vi "Stacking Commnd Sequencer.vi"(4 "Lifter Commands":T2, 5 "Command Series Start Index":i32, 6 "Wait Input":bool=TRUE, 7 "New Command Series":bool=TRUE, 8 "Set Motor Speed":dbl=0.25) -> (0 "Series Finished":bool, 1 "Grabber Solenoid":T1, 2 "Can Solenoid":T1, 3 "Motor Speed":dbl)   [LabVIEW 2014]
doc: "This VI runs a sequence of commands inputed into it. In order to use this properly, it is important to note that:\n -The Sequencer uses the lifter and when it reaches setpoints as the primary method of determining when to move on to another command\n - Currently, giving the lifter two or more identical setpoints in a row WILL cause it to FREEZE. DO NOT INPUT MULTIPLE IDENTICAL SETPOINTS. If you need the lifter to not move for a command, use the NO OP command.\n - The determination of when the command Sequence is completed is when there are four (4) NO OP commands in a row. IF YOU NEED MORE THAN THREE (3) NO OP COMMANDS,SEE ZEUS AND HE WILL CHANGE THE CODE.\n -If there is a wait time for that command, the wait time will OVERRIDE any \"Wait for Input\". In other words, you CANNOT use a WAIT command AND a WAIT TIME command in the same command."
uses:
  <vilib>/Rock Robotics/WPI/Solenoid/WPI_SolenoidValue.ctl
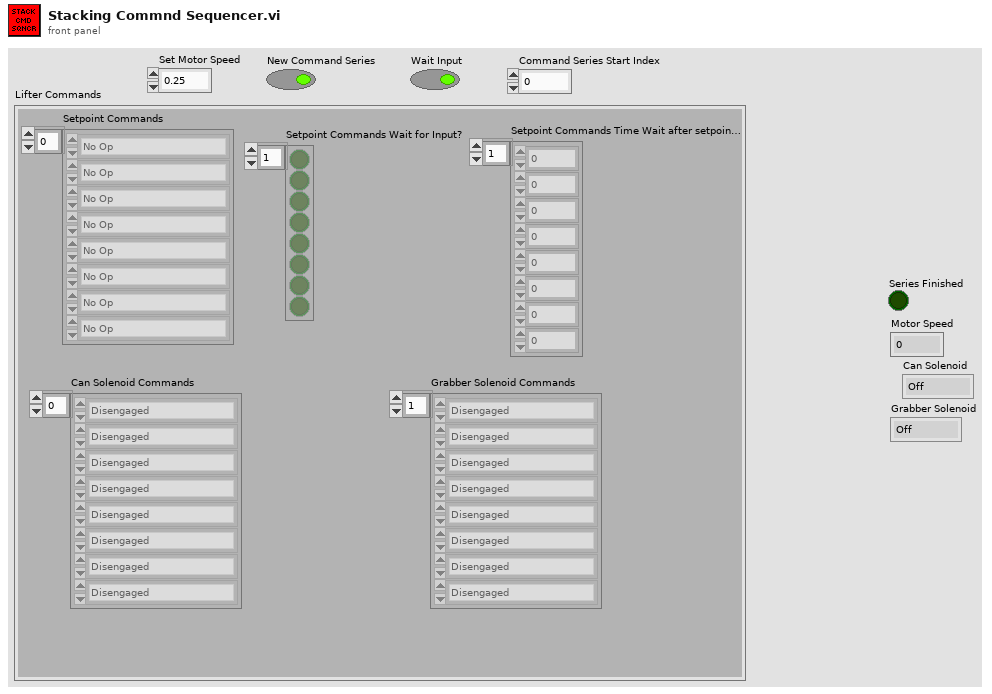
[diagram p1: front panel]
types:
  T1 = typedef "WPI_SolenoidValue.ctl" = enum16{"Off", "On", "Forward", "Reverse"}
  T2 = cluster{"Setpoint Commands":enum16{"No Op", "Setpoint 1", "Setpoint 2", "Setpoint 3", "Setpoint 4", "Setpoint 5"}[], "Setpoint Commands Wait for Input?":bool[], "Setpoint Commands Time Wait after setpoint reachd":i32[], "Can Solenoid Commands":enum16{"Disengaged", "Engaged"}[], "Grabber Solenoid Commands":enum16{"Disengaged", "Engaged"}[]}
  T3 = enum16{"No Op", "Setpoint 1", "Setpoint 2", "Setpoint 3", "Setpoint 4", "Setpoint 5"}[]
  T4 = enum16{"No Op", "Setpoint 1", "Setpoint 2", "Setpoint 3", "Setpoint 4", "Setpoint 5"}
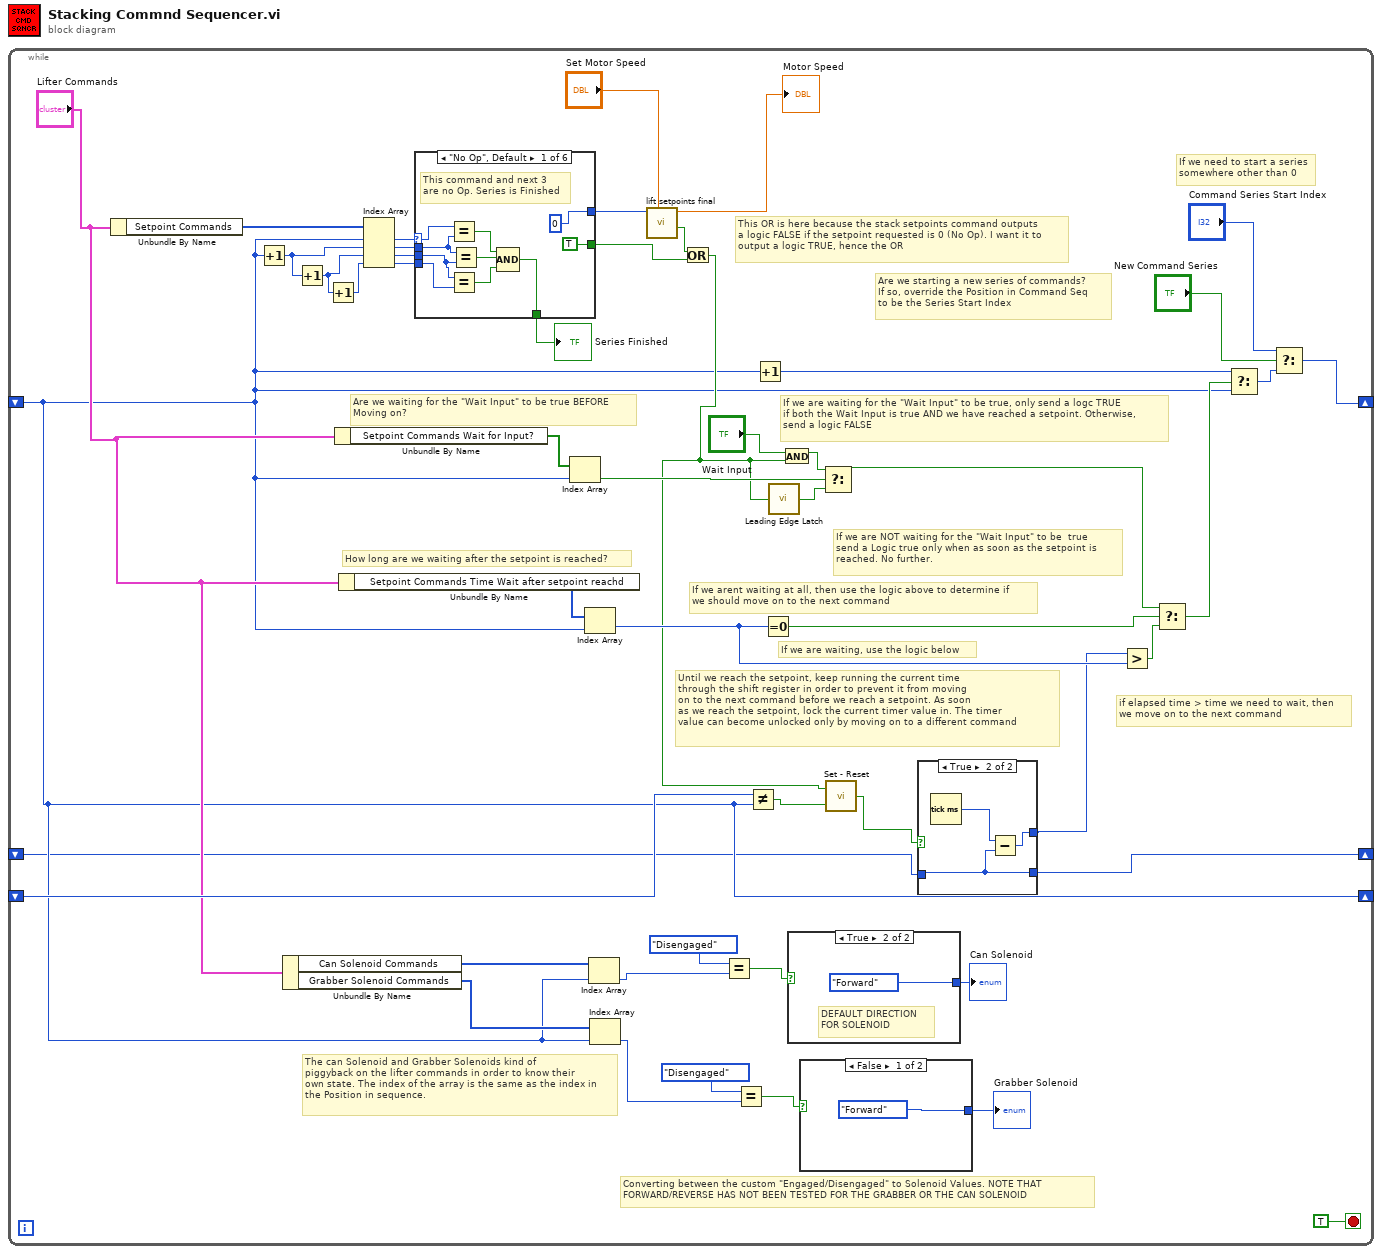
[diagram p0: block diagram]
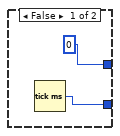
[diagram p2: hidden frame]
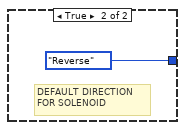
[diagram p3: hidden frame]
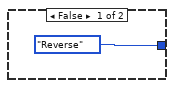
[diagram p4: hidden frame]
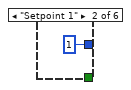
[diagram p5: hidden frame]
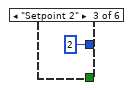
[diagram p6: hidden frame]
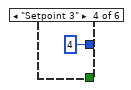
[diagram p7: hidden frame]
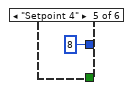
[diagram p8: hidden frame]
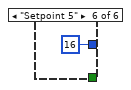
[diagram p9: hidden frame]
diagram:
  n1 = while {
    shift-right: [w32] -> _
    shift-left: _ -> [w10]
    shift-right: [w3] -> _
    shift-left: _ -> [w4]
    shift-right: [w10] -> _
    shift-left: _ -> [w27]
    stop <- TRUE stop-if-true
    # "Converting between the custom \"Engaged/Disengaged\" to Solenoid Values. NOTE THAT \nFORWARD/REVERSE HAS NOT BEEN TESTED FOR THE GRABBER OR THE CAN SOLENOID"
    # "The can Solenoid and Grabber Solenoids kind of\npiggyback on the lifter commands in order to know their\nown state. The index of the array is the same as the index in\nthe Position in sequence."
    # "Are we starting a new series of commands?\nIf so, override the Position in Command Seq\nto be the Series Start Index"
    # "If we need to start a series\nsomewhere other than 0"
    # "if elapsed time > time we need to wait, then\nwe move on to the next command"
    # "If we are waiting, use the logic below"
    # "Until we reach the setpoint, keep running the current time\nthrough the shift register in order to prevent it from moving\non to the next command before we reach a setpoint. As soon\nas we reach the setpoint, lock the current timer value in. The timer\nvalue can become unlocked only by moving on to a different command"
    # "If we arent waiting at all, then use the logic above to determine if \nwe should move on to the next command"
    # "How long are we waiting after the setpoint is reached?"
    # "If we are NOT waiting for the \"Wait Input\" to be  true\nsend a Logic true only when as soon as the setpoint is \nreached. No further."
    # "If we are waiting for the \"Wait Input\" to be true, only send a logc TRUE\nif both the Wait Input is true AND we have reached a setpoint. Otherwise,\nsend a logic FALSE"
    # "Are we waiting for the \"Wait Input\" to be true BEFORE\nMoving on?"
    # "This OR is here because the stack setpoints command outputs\na logic FALSE if the setpoint requested is 0 (No Op). I want it to\noutput a logic TRUE, hence the OR"
    n2 = Unbundle By Name("Lifter Commands") -> ("Setpoint Commands"=w38:T3)
    n3 = Increment(x=w10) -> (x+1=w8:i32)
    n4 = Unbundle By Name("Lifter Commands") -> ("Can Solenoid Commands"=w25:enum16{"Disengaged", "Engaged"}[], "Grabber Solenoid Commands"=w24:enum16{"Disengaged", "Engaged"}[])
    n5 = Increment(x=w8) -> (x+1=w9:i32)
    n6 = Increment(x=w9) -> (x+1=w11:i32)
    n7 = Unbundle By Name("Lifter Commands") -> ("Setpoint Commands Wait for Input?"=w37:bool[])
    n8 = Unbundle By Name("Lifter Commands") -> ("Setpoint Commands Time Wait after setpoint reachd"=w36:i32[])
    n9 = Index Array(array=w38, index #1=w10, index #2=w8, index #3=w9, index #4=w11) -> (element #1=w49:T4, element #2=w15:T4, element #3=w7:T4, element #4=w6:T4)
    n10 = case shown="\"No Op\", Default" w49 {
      selector: w49 -> [w67 _ _ _ _ _]
      tunnel: [0 1 2 4 8 16] -> w43
      tunnel: w15 -> [w66 _ _ _ _ _]
      tunnel: [TRUE _ _ _ _ _] -> w13
      tunnel: w7 -> [w65 _ _ _ _ _]
      tunnel: w6 -> [w64 _ _ _ _ _]
      tunnel: [w60 _ _ _ _ _] -> w5
      frame "No Op", Default {
        # "This command and next 3\nare no Op. Series is Finished"
        n11 = Equal?(x=w67, y=w66) -> (x = y?=w63:bool)
        n12 = Equal?(x=w65, y=w64) -> (x = y?=w61:bool)
        n13 = Equal?(x=w66, y=w65) -> (x = y?=w62:bool)
        n14 = Compound Arithmetic op=AND(w63, w62, w61) -> (w60:bool)
      }
      frame "Setpoint 1" {
      }
      frame "Setpoint 2" {
      }
      frame "Setpoint 3" {
      }
      frame "Setpoint 4" {
      }
      frame "Setpoint 5" {
      }
    }
    "Series Finished" <- w5
    n15 = Index Array(array=w37, index=w10) -> (element=w42:bool)
    n16 = Index Array(array=w36, index=w10) -> (element=w28:i32)
    n17 = Index Array(array=w25, index=w10) -> (element=w23:enum16{"Disengaged", "Engaged"})
    n18 = Index Array(array=w24, index=w10) -> (element=w18:enum16{"Disengaged", "Engaged"})
    n19 = call "lift setpoints final.vi"("Set Motor Speed"="Set Motor Speed", "Requested Position\n(0, 1, 2, 4, 8, 16)"=w43) -> ("Setpoint\nReached"=w14:bool, "Motor Speed"=→"Motor Speed":dbl)  [unwired: 8 in]
    n20 = Or(x=w14, y=w13) -> (x .or. y?=w12:bool)
    n21 = Equal?(x=enum16{"Disengaged", "Engaged"}."Disengaged", y=w23) -> (x = y?=w21:bool)
    n22 = Equal?(x=enum16{"Disengaged", "Engaged"}."Disengaged", y=w18) -> (x = y?=w20:bool)
    n23 = Not Equal?(x=w27, y=w10) -> (x != y?=w31:bool)
    n24 = Increment(x=w10) -> (x+1=w46:i32)
    n25 = Equal To 0?(x=w28) -> (x = 0?=w30:bool)
    n26 = call "Leading Edge Latch.vi"("Input"=w12) -> ("Output"=w33:bool)
    n27 = And(x="Wait Input", y=w12) -> (x .and. y?=w41:bool)
    n28 = case shown="True" w21 {
      tunnel: [WPI_SolenoidValue."Reverse" ("Passive Hooks") WPI_SolenoidValue."Forward" ("Passive Hooks")] -> w17
      frame False {
      }
      frame True {
        # "DEFAULT DIRECTION\nFOR SOLENOID"
      }
    }
    "Can Solenoid" <- w17
    n29 = case shown="False" w20 {
      tunnel: [WPI_SolenoidValue."Forward" ("Passive Hooks") WPI_SolenoidValue."Reverse" ("Passive Hooks")] -> w16
      frame False {
      }
      frame True {
        # "DEFAULT DIRECTION\nFOR SOLENOID"
      }
    }
    "Grabber Solenoid" <- w16
    n30 = Select(t=w41, s=w42, f=w33) -> (s? t:f=w35:bool)
    n31 = call "Set - Reset.vi"("Reset"=w31, "Set"=w12) -> ("Output"=w1:bool)
    n32 = case shown="True" w1 {
      tunnel: [w51 w54] -> w3
      tunnel: w4 -> [_ w54]
      tunnel: [0 w55] -> w2
      frame False {
        n33 = Tick Count (ms)() -> (millisecond timer value=w51:u32)
      }
      frame True {
        n34 = Tick Count (ms)() -> (millisecond timer value=w53:u32)
        n35 = Subtract(x=w53, y=w54) -> (x-y=w55:u32)
      }
    }
    n36 = Greater?(x=w2, y=w28) -> (0:w29:bool)
    n37 = Select(t=w35, s=w30, f=w29) -> (s? t:f=w34:bool)
    n38 = Select(t=w46, s=w34, f=w10) -> (s? t:f=w44:i32)
    n39 = Select(t="Command Series Start Index", s="New Command Series", f=w44) -> (s? t:f=w32:i32)
  }
